vi "ma_Convert Magnitude.vi"(2 "scale":dbl=1.0 format="%0.2f", 3 "conversion":bool, 4 "Array of G in":dbl[](array[numeric]) format="%0.2f", 5 "G in":dbl format="%0.2f") -> (0 "Array G out":dbl[](array[numeric]) format="%0.2f", 1 "G out":dbl format="%0.4f")   [LabVIEW 2020, in "NI_MAPro.lvlib"]
uses:
  NI_MAPro.lvlib
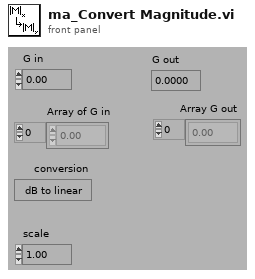
[diagram p1: front panel]
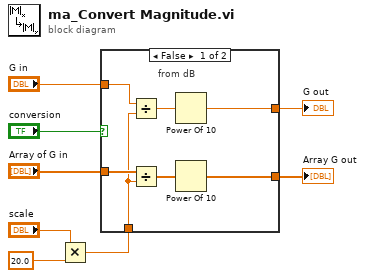
[diagram p0: block diagram]
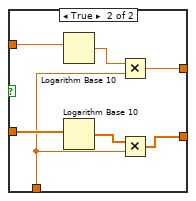
[diagram p2: hidden frame]
diagram:
  n1 = Multiply(x="scale", y=20.0) -> (x*y=w1:dbl)
  n2 = case shown="False" "conversion" {
    tunnel: "G in" -> [w15 w21]
    tunnel: [w13 w20] -> w7
    tunnel: "Array of G in" -> [w11 w18]
    tunnel: [w10 w17] -> w4
    tunnel: w1 -> [w9 w16]
    frame False {
      # "from dB"
      n3 = Divide(x=w15, y=w9) -> (x/y=w14:dbl)
      n4 = Divide(x=w11, y=w9) -> (x/y=w12:dbl[])
      n5 = Power Of 10(x=w14) -> (10^x=w13:dbl)
      n6 = Power Of 10(x=w12) -> (10^x=w10:dbl[])
    }
    frame True {
      n7 = Logarithm Base 10(1:w21) -> (0:w22:dbl)
      n8 = Logarithm Base 10(1:w18) -> (0:w19:dbl[])
      n9 = Multiply(x=w22, y=w16) -> (x*y=w20:dbl)
      n10 = Multiply(x=w19, y=w16) -> (x*y=w17:dbl[])
    }
  }
  "G out" <- w7
  "Array G out" <- w4
